vi "Read Position.vi"(8 "Error In":errorcluster, 11 "SFTP File In":refnum<class "SFTP File.lvclass">) -> (0 "Error Out":errorcluster, 2 "Position":u64, 3 "SFTP File Out":refnum<class "SFTP File.lvclass">)   [LabVIEW 2018, in "Toolkit.lvlib" / "SFTP File.lvclass"]
doc: "Gets the current position in bytes (B) relative to the beginning of the file."
uses:
  SFTP File.lvclass
  SFTP File.lvclass/SFTP File.ctl
  SFTP/SFTP.lvclass/SFTP.ctl
  Session/Session.lvclass/Session.ctl
  SSH/SSH.lvclass/SSH.ctl
  Toolkit.lvlib
  SFTP/SFTP.lvclass
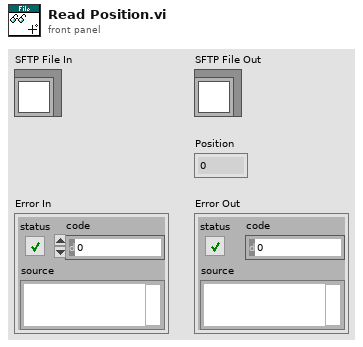
[diagram p1: front panel]
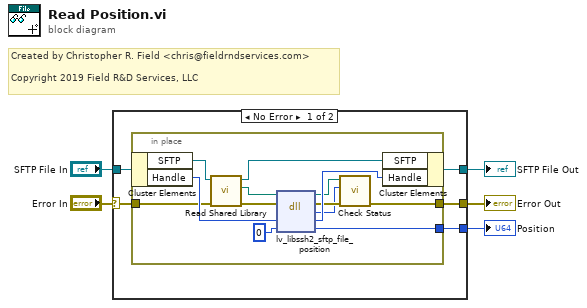
[diagram p0: block diagram]
diagram:
  # "Created by Christopher R. Field <chris@fieldrndservices.com>\n\nCopyright 2019 Field R&D Services, LLC"
  n1 = case shown="No Error" "Error In" {
    selector: "Error In" -> [w9 w24]
    tunnel: "SFTP File In" -> [w10 w25]
    tunnel: [w8 w25] -> w2
    tunnel: [w7 w24] -> w3
    tunnel: [w6 _] -> w1
    frame No Error {
      n2 = in-place {
        in-place-border: w9 -> [w22]
        in-place-border: [w17] -> w7
        in-place-border: [w11] -> w6
        n3 = in-place-cluster #1(w10) -> ("SFTP"=w14:refnum<class "SFTP.lvclass">, "Handle"=w23:u64)
        n4 = call "Read Shared Library.vi"("Error In"=w22, "SFTP In"=w14) -> ("Erorr Out"=w15:errorcluster, "libssh2lv Shared Library"=w12:path, "SFTP Out"=w13:refnum<class "SFTP.lvclass">)  [unwired: 7 in]
        n5 = dll-call lib="libssh2lv.*" fn="lv_libssh2_sftp_file_position"(path in=w12, error in=w15, "handle"=w23, "position"=u64 0 ("read_count")) -> (path out=w19:path, error out=w20:errorcluster, "status"=w18:i32, "handle"=w21:u64, "position"=w11:u64)  [unwired: 1 in]
        n6 = call "Check Status.vi"("Error In"=w20, "Status"=w18, "libssh2lv Shared Library In"=w19) -> ("Error Out"=w17:errorcluster)  [unwired: 7 in, 1 out]
        n7 = in-place-cluster #1("SFTP"=w13, "Handle"=w21) -> (w8:refnum<class "SFTP File.lvclass">)
      }
    }
    frame Error {
    }
  }
  "Error Out" <- w3
  "SFTP File Out" <- w2
  "Position" <- w1
